vi "test Major Frame End.vi"(8 "error in (no error)":errorcluster, 11 "BC Major Frame in":refnum<class "BC Major Frame.lvclass">) -> (0 "error out":errorcluster, 3 "BC Major Frame out":refnum<class "BC Major Frame.lvclass">)   [LabVIEW 2016, in "BC Major Frame.lvclass"]
uses:
  BC Major Frame.lvclass
  Frames & Messages/TypeDefs/BC Op Codes - Verbose.ctl
  Frames & Messages/TypeDefs/BC Condition Codes.ctl
  PPLs/FPGA Interface.lvlibp/FPGA Interface/FPGA Interface.lvclass
  BCI-1553 API.lvlib
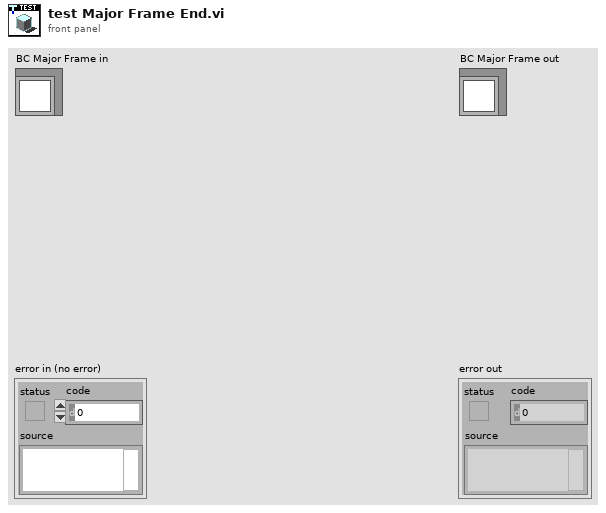
[diagram p1: front panel]
types:
  T1 = typedef "BCI-1553 API.lvlib/BC Op Codes - Verbose.ctl" = enum16{"EXECUTE MSG", "EXECUTE MSG GO", "JUMP", "CALL SUBROUTINE", "RETURN", "INTERRUPT REQUEST", "HALT", "DELAY", "WAIT FRAME TIMER = 0", "COMPARE FRAME TIMER", "COMPARE MSG TIMER", "LOAD TIME TAG CTR", "LOAD TIME TAG CTR HI", "LOAD FRAME TIMER", "START FRAME TIMER", "PUSH TIME TAG COUNT", "PUSH TIME TAG COUNT HI", "PUSH TIME TAG COUNT BOTH", "PUSH BLOCK STATUS WORD", "PUSH CURRENT VALUE", "PUSH INDIRECT", "WAIT EXT TRIGGER", "EXECUTE AND FLIP", "EXECUTE, FLIP, GO", "WRITE VALUE TO WMI", "WRITE VALUE TO MEM", "DECREMENT RAM, SKIP", "FLAG"}
  T2 = typedef "BCI-1553 API.lvlib/BC Condition Codes.ctl" = enum16{"GP0 == 1 || LT", "GP1 == 1 || NE", "GP2 == 1", "GP3 == 1", "GP4 == 1", "GP5 == 1", "GP6 == 1", "GP7 == 1", "NORESP", "FMTERR", "GOODBLOCK", "MSKSTATSET", "BADMSG", "1RETRY", "2RETRY", "ALWAYS"}
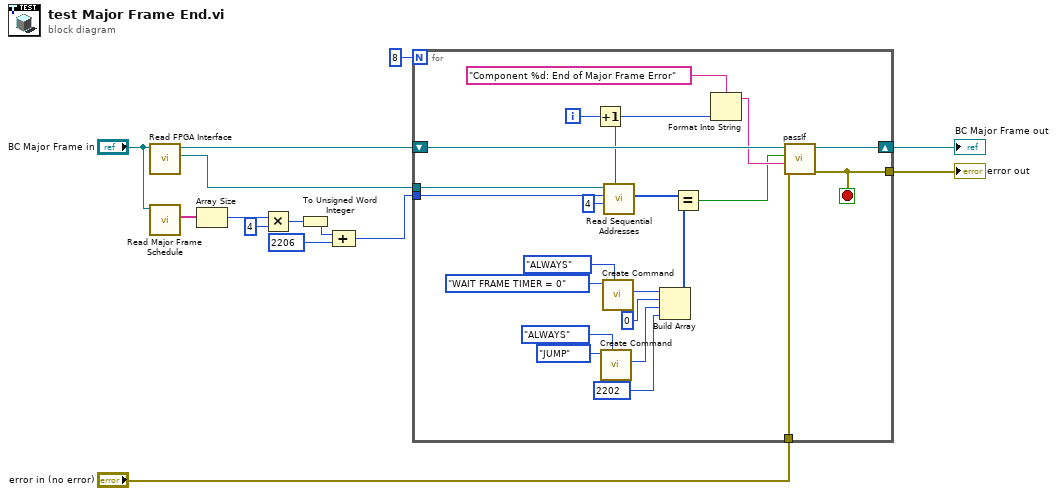
[diagram p0: block diagram]
diagram:
  n1 = call-dynamic "Read FPGA Interface.vi"("1553 Test in"="BC Major Frame in") -> ("FPGA Interface"=w13:refnum<class "FPGA Interface.lvclass">, "1553 Test out"=w14:refnum<class "BC Major Frame.lvclass">)  [unwired: 8 in, 1 out]
  n2 = call-dynamic "Read Major Frame Schedule.vi"("1553 Test in"="BC Major Frame in") -> ("Major Frame Schedule"=w3:string[])  [unwired: 8 in, 2 out]
  n3 = Array Size(array=w3) -> (size(s)=w5:i32)
  n4 = Multiply(x=w5, y=4) -> (x*y=w7:i32)
  n5 = To Unsigned Word Integer(number=w7) -> (unsigned 16bit integer=w8:u16)
  n6 = Compound Arithmetic op=ADD(w8, u16 2206) -> (w1:u16)
  n7 = for {
    N: 8 -> [_]
    shift-right: [w36] -> w11
    shift-left: w14 -> [w35]
    tunnel: w13 -> [w34]
    tunnel: w1 -> [w30]
    tunnel: "error in (no error)" -> [w17]
    tunnel: [w16] -> w10
    i -> [w32]
    stop <- w16 stop-if-true
    n8 = Increment(x=w32) -> (x+1=w28:i32)
    n9 = call "Create Command.vi"("Condition"=BC_Condition_Codes."ALWAYS", "Op Code"=BC_Op_Codes_-_Verbose."JUMP") -> ("Instruction"=w21:u16)  [unwired: 8 in, 1 out]
    n10 = call "Create Command.vi"("Condition"=BC_Condition_Codes."ALWAYS", "Op Code"=BC_Op_Codes_-_Verbose."WAIT FRAME TIMER = 0") -> ("Instruction"=w23:u16)  [unwired: 8 in, 1 out]
    n11 = call-dynamic "Read Sequential Addresses.vi"("Target IC (1-8)"=w28, "Addresses to Read"=u16 4, "Starting Address"=w30, "FPGA Interface in"=w34) -> ("Data"=w19:u16[])  [unwired: 6 in, 1 out]
    n12 = Build Array(w23, u16 0 ("x"), w21, u16 2202) -> (w20:u16[])
    n13 = Equal?(x=w19, y=w20) -> (x = y?=w18:bool)
    n14 = Format Into String(format string="Component %d: End of Major Frame Error" ("custom report message (\"\")"), w28) -> (resulting string=w31:string)  [unwired: 2 in, 1 out]
    n15 = call-dynamic "passIf.vi"("error in (no error)"=w17, "message (\"\")"=w31, "pass"=w18, "TestCase in"=w35) -> ("error out"=w16:errorcluster, "TestCase out"=w36:refnum<class "BC Major Frame.lvclass">)  [unwired: 6 in]
  }
  "error out" <- w10
  "BC Major Frame out" <- w11
